vi "Lognormal Random.vi"(6 "seed":i32=-1, 7 "reset":bool, 9 "c":dbl=1.0, 10 "b":dbl=1.0, 11 "samples":i32=128) -> (0 "error":i32, 3 "Lognormal random numbers":dbl[](array[numeric]))   [LabVIEW 2024, in "NI_Gmath.lvlib"]
doc: "<p>Generates random values from a variate X, where X describes the selected distribution type. You must <a href=\"nihelplauncher://docs/csh?context=lvcore_lvhowto_selectingdefaultinstpolyvi\">manually select the polymorphic instance</a> to use.</p>"
uses:
  NI_Gmath.lvlib
  st_error_code.ctl
panel:
  # "Lognormal Random"
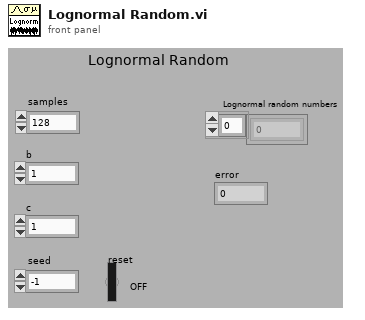
[diagram p1: front panel]
types:
  T1 = typedef "NI_Gmath.lvlib/st_error_code.ctl" = i32
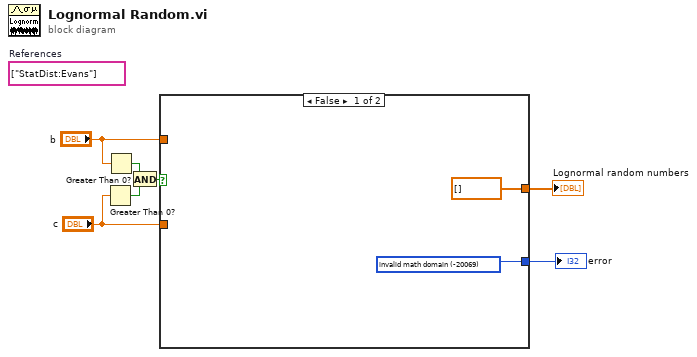
[diagram p0: block diagram]
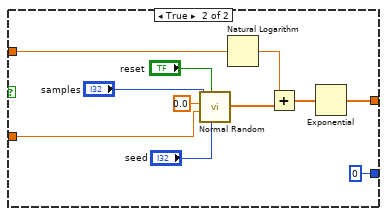
[diagram p2: hidden frame]
diagram:
  (unwired) string[] ["StatDist:Evans"]  # References
  n1 = Greater Than 0?(x="c") -> (x > 0?=w4:bool)
  n2 = Greater Than 0?(x="b") -> (x > 0?=w5:bool)
  n3 = And(x=w5, y=w4) -> (x .and. y?=w1:bool)
  n4 = case shown="False" w1 {
    tunnel: [w8 0 ("invalid math domain")] -> w7
    tunnel: [dbl[] [] w13] -> w6
    tunnel: "b" -> [_ w18]
    tunnel: "c" -> [_ w15]
    frame False {
      w8 = T1 -20069 items=["invalid math domain"=-20069, "Fourier interpolation size m >= n"=-20070, "empty array"=-20003] ("stat interp error code")
    }
    frame True {
      n5 = call "Normal Random.vi"("seed"="seed", "reset"="reset", "std"=w15, "mean"=0.0, "samples"="samples") -> ("normal random data"=w14:dbl[])  [unwired: 5 in, 1 out]
      n6 = Natural Logarithm(1:w18) -> (0:w19:dbl)
      n7 = Add(x=w19, y=w14) -> (x+y=w20:dbl[])
      n8 = Exponential(1:w20) -> (0:w13:dbl[])
    }
  }
  "error" <- w7
  "Lognormal random numbers" <- w6
